vi "AudioStreamer.Set Params.vi"(7 "Masker":T1) -> (15 "error out":errorcluster)   [LabVIEW 2020]
uses:
  Typedefs/NoiseGenerator.Params.ctl
  SubVIs/NoiseGenerator.Globals.vi
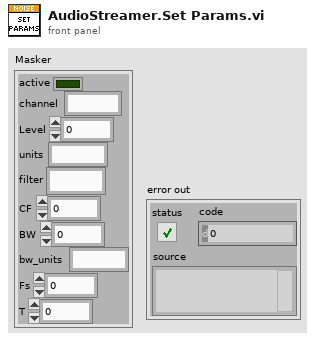
[diagram p1: front panel]
types:
  T1 = typedef "NoiseGenerator.Params.ctl" = cluster{"active":bool, "channel":string, "Level":dbl, "units":string, "filter":string, "CF":dbl, "BW":dbl, "bw_units":string, "Fs":dbl, "T":dbl}
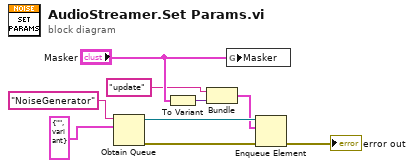
[diagram p0: block diagram]
diagram:
  n1 = Obtain Queue(name (unnamed)="NoiseGenerator", element data type=cluster{string, variant} {"", variant}) -> (queue out=w6:refnum<queue>, error out=w7:errorcluster)  [unwired: 3 in, 1 out]
  n2 = To Variant(anything="Masker") -> (Variant=w3:variant)
  n3 = Bundle("update", "Variant"=w3) -> (w1:cluster{string, "Variant":variant})  [unwired: 1 in]
  n4 = global write "NoiseGenerator.Globals.vi" "Masker"("Masker") -> ()
  n5 = Enqueue Element(queue=w6, element=w1, error in (no error)=w7) -> (error out=→"error out":errorcluster)  [unwired: 1 in, 2 out]
